vi "Live_ConvertSettings_Example_IMAQ.vi"() -> ()   [LabVIEW 2019]
doc: "This example demonstrates the image acquisition with one camera in ring buffer mode together with a live display of the latest images during record. After record is stopped, the images can be addressed by index.\nAdditionally the image convert settings can be adjusted at any time\nNote that this example will not be fail save, i.e. doesnt react on errors, just handles them forward to the end\n\nUsage:\nSelect your required image count and the camera setup before you start the program.\nOnce started, the camera class will be initialized and images will be recorded and displayed automatically\nYou can stop the images by pressing stop record.\nAfter stopped, the image at the selected index will be read out\nTo finish the program click on quit application, this will force an exit of the camera class\nYou can change your required ROI after and also during the record."
uses:
  camera/Camera.lvclass
  pco.sdk/TimingControl/TimingControl.lvlib
panel:
  in  "settingsChanged":bool
  in  "Trigger":bool
  in  "LUT File":path
  in  "data_format":T1(ring)=enum."RGBA8"
  out "Image":T2(plugin-control)
  in  "Auto Range":bool
  out "rawImage":u16[][](array[numeric])
  in  "iContrast [%]":i32 min=-100 max=99 step=1
  in  "Gamma":dbl=1.0 min=0.01 max=10.0 step=0.01 format="%.2f"
  in  "whiteBalance":bool
  in  "iScale_max":u16=60000 step=1
  in  "iScale_min":u16=200 step=1
  in  "Image Index":u32 max=9
  out "Recorded Images":u32
  in  "TriggerMode":T3(ring)
  in  "Quit":bool
  out "Error":errorcluster {"code" format="%x"}
  in  "Stop Record":bool
  out "Recording On":bool
  in  "cropY1":u64=2 min=1 max=2160 step=1
  in  "cropX1":u64=2 min=1 max=2560 step=1
  in  "cropY0":u64=1 min=1 max=2159 step=1
  in  "cropX0":u64=1 min=1 max=2559 step=1
  out "Image Height":u64
  out "Image Width":u64
  in  "dwImgCount":u32=10 caption="Required Number of Images" max=2397
  in  "Exposure Time [s]":dbl=0.010000000000000002 min=0.0005 max=2.0 step=0.001
  # "This example demonstrates the image acquisition with one camera in ring buffer mode together with a live display of the latest images during record. After record is stopped, the images can be addressed by index.\nAdditionally the image convert settings can be adjusted at any time\nNote that this example will not be fail save, i.e. doesnt react on errors, just handles them forward to the end\n\nUsage:\nSelect your required image count and the camera setup before you start the program.\nOnce started, the camera class will be initialized and images will be recorded and displayed automatically\nYou can stop the images by pressing stop record.\nAfter stopped, the image at the selected index will be read out\nTo finish the program click on quit application, this will force an exit of the camera class\nYou can change the cropped region after and also during the record."
  # "pco.labview"
  # "Camera Setup"
  # "Recording Control"
  # "Parameters for image readout"
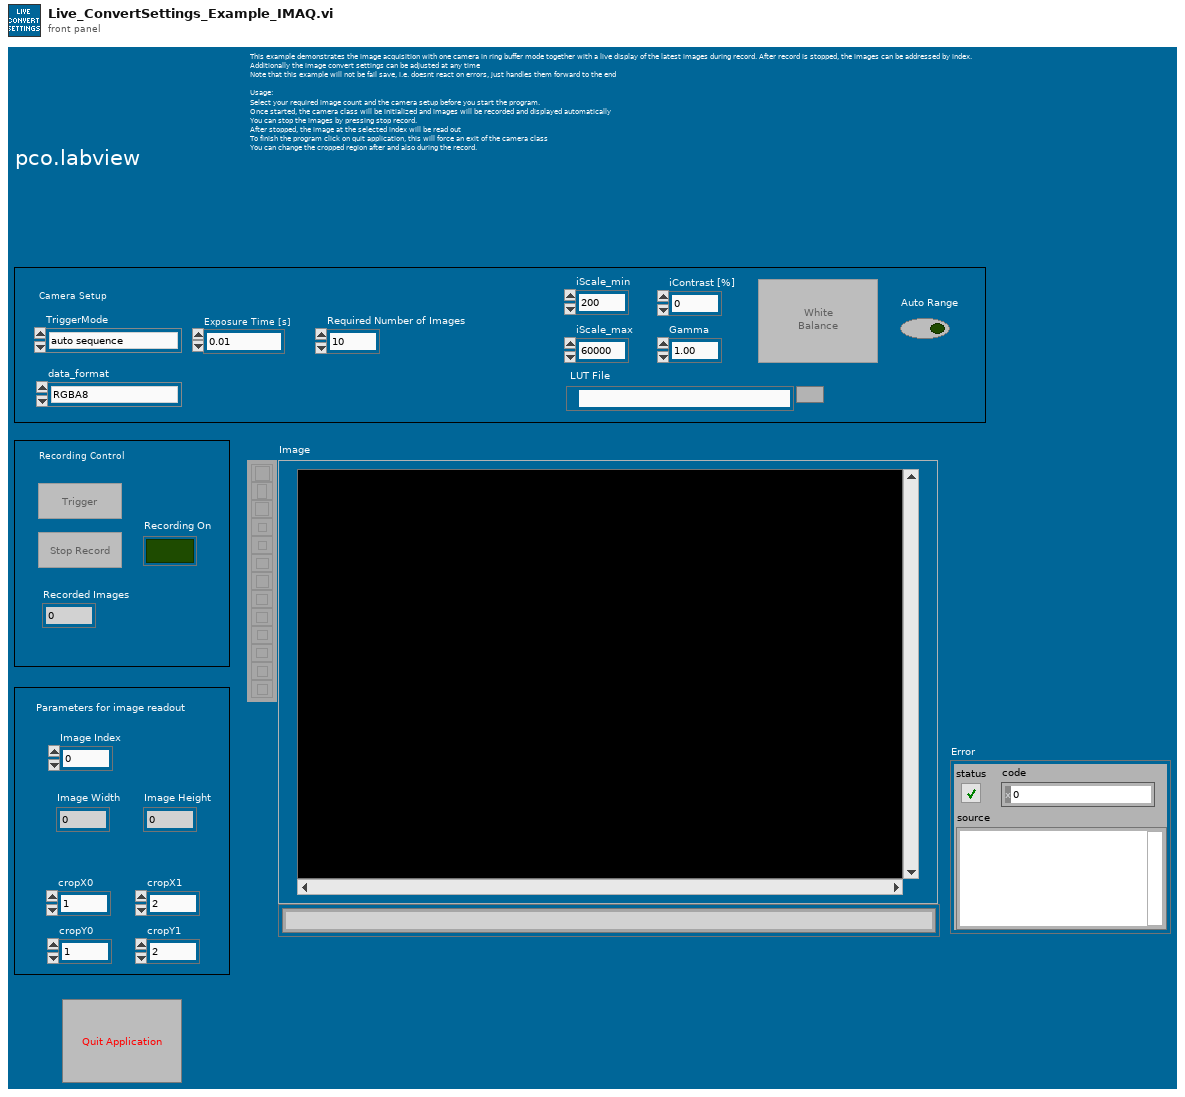
[diagram p1: front panel]
types:
  T1 = enum16{"Undefined", "Mono8", "Mono16", "BGRA8", "RGBA8", "BGRA16", "RGBA16", "CompressedMono8"}
  T2 = typedef "IMAQ Image.ctl" = refnum<image>
  T3 = enum16{"auto sequence", "software trigger", "external exposure start", "external exposure control"}
  T4 = enum16{"sequence", "sequence non blocking", "ring buffer", "fifo", "tif", "multitif", "pcoraw", "b16", "dicom", "multidicom", "camram_ring", "camram_segment"}
  T5 = enum8{"Enabled", "Disabled", "Disabled and Grayed Out"}
  T6 = cluster{"serial":u32, "type":u16, "sub_type":u16, "interface_type":u16, "bit_resolution":u16, "min_exposure_time_s":dbl, "max_exposure_time_s":dbl, "min_exposure_step_s":dbl, "min_delay_time_s":dbl, "max_delay_time_s":dbl, "min_delay_step_s":dbl, "min_width":u64, "min_height":u64, "max_width":u64, "max_height":u64, "roi_step_horz":u64, "roi_step_vert":u64, "roi_symmetric_horz":bool, "roi_symmetric_vert":bool, "has_timestamp_mode":bool, "has_timestamp_mode_ascii_only":bool, "pixelrate_vec":u32[], "conversion_factor_vec":sgl[], "has_trigger_mode_extexpctrl":bool, "has_acquire_mode":bool, "has_ext_acquire_mode":bool, "has_metadata_mode":bool, "has_ram":bool, "binning_horz_vec":u16[], "binning_vert_vec":u16[], "has_average_binning":bool, "pixel_format_vec":u32[]}
  T7 = typedef "Image Type" = u32
  T8 = cluster{"wSignalNum":u16, "wEnabled":u16, "wType":u16, "wPolarity":u16, "wFilterSetting":u16, "wSelected":u16, "dwParameter":u32[], "dwSignalFunctionality":u32[]}
  T9 = typedef "Camera.lvclass/binning.ctl" = cluster{"vert":u16, "horz":u16, "mode":u16}
  T10 = cluster{"exposure_time_s":dbl, "delay_time_s":dbl, "roi":cluster{"x0":u64, "y0":u64, "x1":u64, "y1":u64}, "timestamp_mode":u16, "pixelrate":u32, "conversion_factor":sgl, "trigger_mode":u16, "acquire_mode":u16, "acquire_sequence_number":u32, "metadata_mode":u16, "noisefilter_mode":u16, "pixel_format":u32, "binning":T9, "auto_exposure":cluster{"region":u16, "min_exposure_s":dbl, "max_exposure_s":dbl}}
  T11 = cluster{"sharpen":bool, "adaptive_sharpen":bool, "flip_vertical":bool, "auto_minmax":bool, "add_conv_flags":u32, "min_limit":u16, "max_limit":u16, "gamma":dbl, "contrast":i32, "pco_debayer_algorithm":bool, "color_temperature":i32, "color_saturation":i32, "color_vibrance":i32, "color_tint":i32, "lut_file":path}
  T12 = cluster{"Plane 4 (alpha)":u16, "Plane 1 (Red)":u16, "Plane 2 (Green)":u16, "Plane 3 (Blue)":u16}[][]
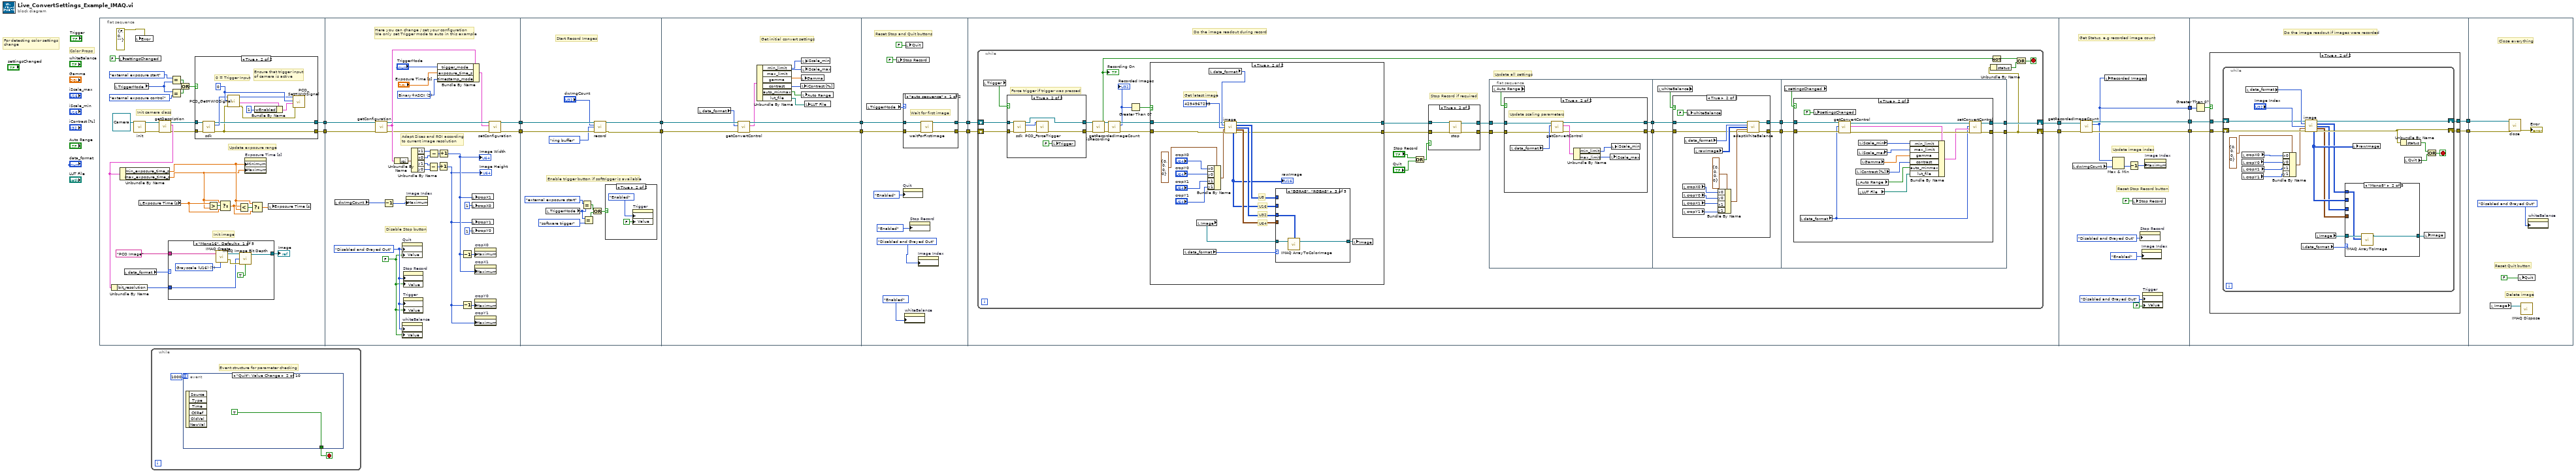
[diagram p0: block diagram]
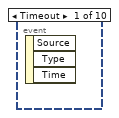
[diagram p2: hidden frame]
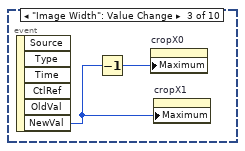
[diagram p3: hidden frame]
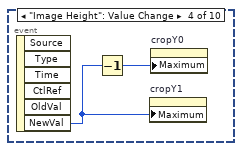
[diagram p4: hidden frame]
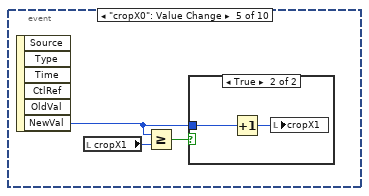
[diagram p5: hidden frame]
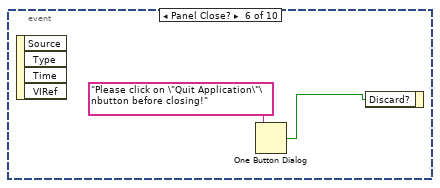
[diagram p7: hidden frame]
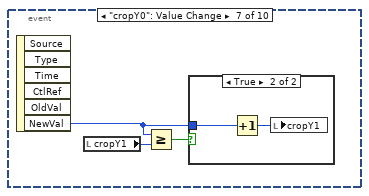
[diagram p8: hidden frame]
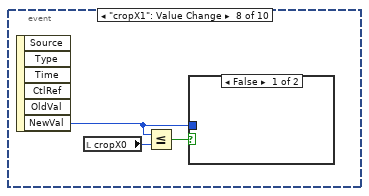
[diagram p10: hidden frame]
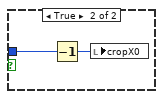
[diagram p11: hidden frame]
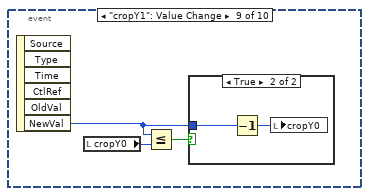
[diagram p12: hidden frame]
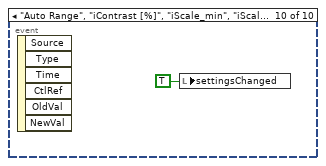
[diagram p14: hidden frame]
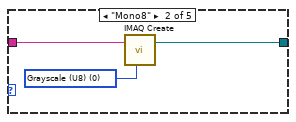
[diagram p16: hidden frame]
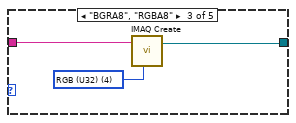
[diagram p17: hidden frame]
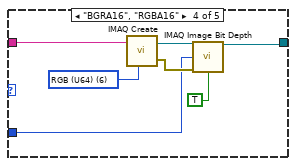
[diagram p18: hidden frame]
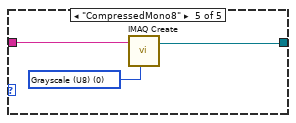
[diagram p19: hidden frame]
diagram:
  # "For detecting color settings\nchange"
  # "Color Props"
  n1 = flat-sequence {
    tunnel: [w24] -> w7
    tunnel: [w25] -> w1
    tunnel: [w85] -> w17
    tunnel: [w89] -> w16
    tunnel: w7 -> [w84]
    tunnel: w1 -> [w83]
    tunnel: w17 -> [w119]
    tunnel: w16 -> [w120]
    tunnel: [w116] -> w11
    tunnel: [w117] -> w8
    tunnel: w11 -> [w133]
    tunnel: [w128] -> w10
    tunnel: [w134] -> w9
    tunnel: w8 -> [w124]
    tunnel: w10 -> [w141]
    tunnel: w9 -> [w142]
    tunnel: [w140] -> w15
    tunnel: [w137] -> w3
    tunnel: w15 -> [w155]
    tunnel: [w154] -> w14
    tunnel: [w153] -> w6
    tunnel: w3 -> [w152]
    tunnel: w14 -> [w302]
    tunnel: [w300] -> w13
    tunnel: w6 -> [w295]
    tunnel: [w294] -> w5
    tunnel: [w293] -> w2
    tunnel: w13 -> [w311]
    tunnel: [w310] -> w12
    tunnel: w5 -> [w309]
    tunnel: [w308] -> w4
    tunnel: w2 -> [w306]
    tunnel: w12 -> [w359]
    tunnel: w4 -> [w356]
    frame #0 {
      # "Update exposure range"
      # "Init image"
      # "Init camera class"
      n2 = local read "TriggerMode"() -> (w18:T3)
      n3 = local write "settingsChanged"(FALSE ("settingsChanged")) -> ()
      n4 = local read "data_format"() -> (w31:T1)
      n5 = call-dynamic "init.vi"("Camera in"=refnum<class "Camera.lvclass"> refnum) -> ("Camera out"=w34:refnum<class "Camera.lvclass">, "error out"=w35:errorcluster)  [unwired: 8 in]
      n6 = local write "Error"(errorcluster {"status"=FALSE, "code"=0, "source"=""} ("error IO")) -> ()
      n7 = local read "Exposure Time [s]"() -> (w43:dbl)
      n8 = call-dynamic "getDescription.vi"("error in (no error)"=w35, "Camera in"=w34) -> ("error out"=w26:errorcluster, "description"=w29:T6, "Camera out"=w27:refnum<class "Camera.lvclass">)  [unwired: 7 in]
      n9 = Unbundle By Name(w29) -> ("bit_resolution"=w28:u16)
      n10 = Unbundle By Name(w29) -> ("min_exposure_time_s"=w33:dbl, "max_exposure_time_s"=w32:dbl)
      n11 = case shown="\"Mono16\", Default" w31 {
        tunnel: "PCO Image" ("Image Name") -> [w63 w67 w69 w76 w79]
        tunnel: [w59 w65 w68 w72 w78] -> w36
        tunnel: w28 -> [w58 _ _ w71 _]
        frame "Mono16", Default {
          w64 = T7 7 items=["Grayscale (U8)", "Grayscale (I16)", "Grayscale (SGL)", "Complex (CSG)", "RGB (U32)", "HSL (U32)", "RGB (U64)", "Grayscale (U16)"] ("Image Type")
          n12 = call "IMAQ Create"("Image Name"=w63, "Image Type"=w64) -> ("New Image"=w61:T2, "error out"=w60:errorcluster)  [unwired: 3 in]
          n13 = call "IMAQ Image Bit Depth"("Image"=w61, "Bit Depth (0)"=w58, "error in (no error)"=w60, "Get/Set Bit Depth? (Set)"=TRUE) -> ("Image Out"=w59:T2)  [unwired: 9 in, 2 out]
        }
        frame "Mono8" {
          w66 = T7 0 items=["Grayscale (U8)", "Grayscale (I16)", "Grayscale (SGL)", "Complex (CSG)", "RGB (U32)", "HSL (U32)", "RGB (U64)", "Grayscale (U16)"] ("Image Type")
          n14 = call "IMAQ Create"("Image Name"=w67, "Image Type"=w66) -> ("New Image"=w65:T2)  [unwired: 3 in, 1 out]
        }
        frame "BGRA8", "RGBA8" {
          w70 = T7 4 items=["Grayscale (U8)", "Grayscale (I16)", "Grayscale (SGL)", "Complex (CSG)", "RGB (U32)", "HSL (U32)", "RGB (U64)", "Grayscale (U16)"] ("Image Type")
          n15 = call "IMAQ Create"("Image Name"=w69, "Image Type"=w70) -> ("New Image"=w68:T2)  [unwired: 3 in, 1 out]
        }
        frame "BGRA16", "RGBA16" {
          w77 = T7 6 items=["Grayscale (U8)", "Grayscale (I16)", "Grayscale (SGL)", "Complex (CSG)", "RGB (U32)", "HSL (U32)", "RGB (U64)", "Grayscale (U16)"] ("Image Type")
          n16 = call "IMAQ Create"("Image Name"=w76, "Image Type"=w77) -> ("New Image"=w74:T2, "error out"=w73:errorcluster)  [unwired: 3 in]
          n17 = call "IMAQ Image Bit Depth"("Image"=w74, "Bit Depth (0)"=w71, "error in (no error)"=w73, "Get/Set Bit Depth? (Set)"=TRUE) -> ("Image Out"=w72:T2)  [unwired: 9 in, 2 out]
        }
        frame "CompressedMono8" {
          w80 = T7 0 items=["Grayscale (U8)", "Grayscale (I16)", "Grayscale (SGL)", "Complex (CSG)", "RGB (U32)", "HSL (U32)", "RGB (U64)", "Grayscale (U16)"] ("Image Type")
          n18 = call "IMAQ Create"("Image Name"=w79, "Image Type"=w80) -> ("New Image"=w78:T2)  [unwired: 3 in, 1 out]
        }
      }
      "Image" <- w36
      n19 = Equal?(x=T3."external exposure start" ("TriggerMode"), y=w18) -> (x = y?=w22:bool)
      n20 = Equal?(x=w18, y=T3."external exposure control" ("TriggerMode")) -> (x = y?=w21:bool)
      n21 = Or(x=w22, y=w21) -> (x .or. y?=w20:bool)
      n22 = case shown="True" w20 {
        tunnel: w27 -> [w46 w50]
        tunnel: w26 -> [w45 w49]
        tunnel: [w45 w47] -> w25
        tunnel: [w46 w48] -> w24
        frame False {
        }
        frame True {
          w55 = u16 0 ("wSignalNum")
          # "0 = Trigger Input"
          # "Ensure that trigger input\nof camera is active"
          n23 = call-dynamic "sdk.vi"("Camera in"=w50, "error in (no error)"=w49) -> ("Camera out"=w48:refnum<class "Camera.lvclass">, "sdk"=w51:u64, "error out"=w47:errorcluster)  [unwired: 11 in]
          n24 = call "PCO_GetHWIOSignal.vi"("error in (no error)"=w47, "wSignalNum"=w55, "ph"=w51) -> ("error out"=w53:errorcluster, "strSignal"=w57:T8, "ph out"=w52:u64)  [unwired: 5 in, 1 out]
          n25 = Bundle By Name(cluster=w57, "wEnabled"=u16 1) -> (w54:T8)
          n26 = call "PCO_SetHWIOSignal.vi"("error in (no error)"=w53, "strSignal"=w54, "wSignalNum"=w55, "ph"=w52) -> ()  [unwired: 5 in, 3 out]
        }
      }
      n27 = Greater?(x=w43, y=w32) -> (0:w44:bool)
      n28 = Select(t=w32, s=w44, f=w43) -> (s? t:f=w41:dbl)
      n29 = Less?(x=w41, y=w33) -> (x < y?=w42:bool)
      n30 = property on="Exposure Time [s]" class="DigNum (strict)"("Minimum"=w33, "Maximum"=w32) -> ()  [unwired: 2 in, 2 out]
      n31 = Select(t=w33, s=w42, f=w41) -> (s? t:f=w40:dbl)
      n32 = local write "Exposure Time [s]"(w40) -> ()
    }
    frame #1 {
      w95 = u16 2 items=["OFF", "Binary", "Binary+ASCII", "ASCII"] ("wTimeStampMode")
      w81 = FALSE ("Stop")
      w82 = T5."Disabled and Grayed Out" ("Disabled")
      # "Disable Stop button"
      # "Adapt Sizes and ROI according\nto current image resolution"
      # "Here you can change / set your configuration\nWe only set Trigger mode to auto in this example"
      n33 = local read "dwImgCount"() -> (w96:u32)
      n34 = call-dynamic "getConfiguration.vi"("error in (no error)"=w83, "Camera in"=w84) -> ("error out"=w90:errorcluster, "configuration"=w101:T10, "Camera out"=w92:refnum<class "Camera.lvclass">)  [unwired: 7 in]
      n35 = Decrement(x=w96) -> (x-1=w86:u32)
      n36 = Unbundle By Name(w101) -> ("roi"=w102:cluster{"x0":u64, "y0":u64, "x1":u64, "y1":u64})
      n37 = property on="Quit" class="Bool (strict)"("DisabledEnum"=w82, "Value"=w81) -> ()  [unwired: 2 in, 2 out]
      n38 = property on="whiteBalance" class="Bool (strict)"("DisabledEnum"=w82, "Value"=w81) -> ()  [unwired: 2 in, 2 out]
      n39 = property on="Stop Record" class="Bool (strict)"("DisabledEnum"=w82, "Value"=w81) -> ()  [unwired: 2 in, 2 out]
      n40 = property on="Trigger" class="Bool (strict)"("DisabledEnum"=w82, "Value"=w81) -> ()  [unwired: 2 in, 2 out]
      n41 = property on="Image Index" class="DigNum (strict)"("Maximum"=w86) -> ()  [unwired: 2 in, 2 out]
      n42 = Unbundle By Name(w102) -> ("x1"=w104:u64, "x0"=w103:u64, "y1"=w106:u64, "y0"=w105:u64)
      n43 = Subtract(x=w106, y=w105) -> (x-y=w108:u64)
      n44 = Subtract(x=w104, y=w103) -> (x-y=w107:u64)
      n45 = Bundle By Name(cluster=w101, "trigger_mode"="TriggerMode", "exposure_time_s"="Exposure Time [s]", "timestamp_mode"=w95) -> (w91:T10)
      n46 = Increment(x=w108) -> (x+1=w87:u64)
      "Image Height" <- w87
      n47 = Increment(x=w107) -> (x+1=w88:u64)
      "Image Width" <- w88
      n48 = Decrement(x=w88) -> (x-1=w99:u64)
      n49 = Decrement(x=w87) -> (x-1=w100:u64)
      n50 = local write "cropX1"(w88) -> ()
      n51 = local write "cropX0"(u64 1 ("roiY0")) -> ()
      n52 = local write "cropY1"(w87) -> ()
      n53 = local write "cropY0"(u64 1 ("roiY0")) -> ()
      n54 = property on="cropX0" class="DigNum (strict)"("Maximum"=w99) -> ()  [unwired: 2 in, 2 out]
      n55 = property on="cropX1" class="DigNum (strict)"("Maximum"=w88) -> ()  [unwired: 2 in, 2 out]
      n56 = property on="cropY0" class="DigNum (strict)"("Maximum"=w100) -> ()  [unwired: 2 in, 2 out]
      n57 = property on="cropY1" class="DigNum (strict)"("Maximum"=w87) -> ()  [unwired: 2 in, 2 out]
      n58 = call-dynamic "setConfiguration.vi"("error in (no error)"=w90, "configuration"=w91, "Camera in"=w92) -> ("error out"=w89:errorcluster, "Camera out"=w85:refnum<class "Camera.lvclass">)  [unwired: 7 in]
    }
    frame #2 {
      # "Enable trigger button if softtrigger is available"
      # "Start Record Images"
      n59 = local read "TriggerMode"() -> (w114:T3)
      n60 = Equal?(x=T3."external exposure start" ("TriggerMode"), y=w114) -> (x = y?=w111:bool)
      n61 = Equal?(x=w114, y=T3."software trigger" ("TriggerMode")) -> (x = y?=w110:bool)
      n62 = Or(x=w111, y=w110) -> (x .or. y?=w112:bool)
      n63 = call-dynamic "record.vi"("Camera in"=w119, "num_images"="dwImgCount", "record_mode"=T4."ring buffer", "error in (no error)"=w120) -> ("Camera out"=w117:refnum<class "Camera.lvclass">, "error out"=w116:errorcluster)  [unwired: 10 in]
      n64 = case shown="True" w112 {
        frame False {
        }
        frame True {
          n65 = property on="Trigger" class="Bool (strict)"("DisabledEnum"=T5."Enabled" ("Disabled"), "Value"=FALSE ("Trigger")) -> ()  [unwired: 2 in, 2 out]
        }
      }
    }
    frame #3 {
      # "Get initial convert settings"
      n66 = local read "data_format"() -> (w123:T1)
      n67 = call-dynamic "getConvertControl.vi"("error in (no error)"=w133, "data_format"=w123, "Camera in"=w124) -> ("error out"=w128:errorcluster, "convert_control"=w132:T11, "Camera out"=w134:refnum<class "Camera.lvclass">)  [unwired: 6 in]
      n68 = Unbundle By Name(w132) -> ("min_limit"=w130:u16, "max_limit"=w129:u16, "gamma"=w131:dbl, "contrast"=w127:i32, "auto_minmax"=w126:bool, "lut_file"=w125:path)
      n69 = local write "iContrast [%]"(w127) -> ()
      n70 = local write "Gamma"(w131) -> ()
      n71 = local write "iScale_min"(w130) -> ()
      n72 = local write "iScale_max"(w129) -> ()
      n73 = local write "Auto Range"(w126) -> ()
      n74 = local write "LUT File"(w125) -> ()
    }
    frame #4 {
      # "Reset Stop and Quit buttons"
      n75 = local read "TriggerMode"() -> (w135:T3)
      n76 = local write "Stop Record"(FALSE ("Stop Record")) -> ()
      n77 = case shown="\"auto sequence\"" w135 {
        tunnel: w142 -> [w149 w151]
        tunnel: w141 -> [w148 w150]
        tunnel: [w147 w150] -> w140
        tunnel: [w146 w151] -> w137
        frame "auto sequence" {
          # "Wait for first image"
          n78 = call-dynamic "waitForFirstImage.vi"("error in (no error)"=w148, "Camera in"=w149) -> ("error out"=w147:errorcluster, "Camera out"=w146:refnum<class "Camera.lvclass">)  [unwired: 8 in]
        }
        frame Default {
          # "Don't wait \nif we trigger"
        }
      }
      n79 = property on="Quit" class="Bool (strict)"("DisabledEnum"=T5."Enabled" ("Disabled")) -> ()  [unwired: 2 in, 2 out]
      n80 = property on="whiteBalance" class="Bool (strict)"("DisabledEnum"=T5."Enabled" ("Disabled")) -> ()  [unwired: 2 in, 2 out]
      n81 = local write "Quit"(FALSE ("Stop")) -> ()
      n82 = property on="Stop Record" class="Bool (strict)"("DisabledEnum"=T5."Enabled" ("Disabled")) -> ()  [unwired: 2 in, 2 out]
      n83 = property on="Image Index" class="DigNum (strict)"("DisabledEnum"=T5."Disabled and Grayed Out" ("Disabled")) -> ()  [unwired: 2 in, 2 out]
    }
    frame #5 {
      # "Do the image readout during record"
      n84 = while {
        shift-right: [w165] -> w154
        shift-left: w155 -> [w168]
        shift-right: [w171] -> w153
        shift-left: w152 -> [w169]
        stop <- w183 stop-if-true
        # "Stop Record if required"
        # "Force trigger if trigger was pressed"
        # "Update all settings"
        n85 = local read "Trigger"() -> (w170:bool)
        n86 = case shown="True" w170 {
          tunnel: w169 -> [w227 w232]
          tunnel: w168 -> [w226 w231]
          tunnel: [w227 w230] -> w167
          tunnel: [w226 w229] -> w166
          frame False {
          }
          frame True {
            n87 = call-dynamic "sdk.vi"("Camera in"=w232, "error in (no error)"=w231) -> ("Camera out"=w230:refnum<class "Camera.lvclass">, "sdk"=w233:u64, "error out"=w234:errorcluster)  [unwired: 11 in]
            n88 = call "PCO_ForceTrigger.vi"("error in (no error)"=w234, "ph"=w233) -> ("error out"=w229:errorcluster)  [unwired: 6 in, 3 out]
            n89 = local write "Trigger"(FALSE ("Trigger")) -> ()
          }
        }
        n90 = call-dynamic "isRecording.vi"("Camera in"=w167, "error in (no error)"=w166) -> ("Camera out"=w179:refnum<class "Camera.lvclass">, "recording"=w181:bool, "error out"=w178:errorcluster)  [unwired: 11 in]
        "Recording On" <- w181
        n91 = call-dynamic "getRecordedImageCount.vi"("Camera in"=w179, "error in (no error)"=w178) -> ("Camera out"=w176:refnum<class "Camera.lvclass">, "recorded_image_count"=w164:u32, "error out"=w177:errorcluster)  [unwired: 11 in]
        "Recorded Images" <- w164
        n92 = Greater Than 0?(x=w164) -> (x > 0?=w163:bool)
        n93 = case shown="True" w163 {
          tunnel: w177 -> [w190 w203]
          tunnel: w176 -> [w191 w194]
          tunnel: [w190 w192] -> w159
          tunnel: [w191 w193] -> w158
          frame False {
          }
          frame True {
            # "U64"
            # "U32"
            # "U8"
            # "U16"
            # "Get latest image"
            n94 = local read "data_format"() -> (w195:T1)
            n95 = local read "Image"() -> (w200:T2)
            n96 = Bundle By Name(cluster=cluster{"x0":u64, "y0":u64, "x1":u64, "y1":u64} {"x0"=0, "y0"=0, "x1"=0, "y1"=0} ("roi"), "x0"="cropX0", "y0"="cropY0", "x1"="cropX1", "y1"="cropY1") -> (w206:cluster{"x0":u64, "y0":u64, "x1":u64, "y1":u64})
            n97 = local read "data_format"() -> (w202:T1)
            n98 = call-dynamic "image.vi"("Camera in"=w194, "data_format"=w202, "image_index"=u32 4294967295 ("dwImgIdx"), "crop"=w206, "error in (no error)"=w203) -> ("Camera out"=w193:refnum<class "Camera.lvclass">, "image (U8)"=w197:u8[][], "image (U32)"=w198:u32[][], "image (U64)"=w199:T12, "raw_image (U16)"=w196:u16[][], "error out"=w192:errorcluster)  [unwired: 2 in, 3 out]
            "rawImage" <- w196
            n99 = case shown="\"BGRA8\", \"RGBA8\"" w195 {
              tunnel: w200 -> [w213 w216 w219 w222 w225]
              tunnel: [w211 w214 w218 w220 w224] -> w201
              tunnel: w199 -> [_ _ _ w221 _]
              tunnel: w198 -> [_ _ w217 _ _]
              tunnel: w197 -> [_ w215 _ _ w223]
              tunnel: w196 -> [w212 _ _ _ _]
              frame "Mono16", Default {
                n100 = call "IMAQ ArrayToImage"("Image Pixels (U16)"=w212, "Image"=w213) -> ("Image Out"=w211:T2)  [unwired: 8 in, 1 out]
              }
              frame "Mono8" {
                n101 = call "IMAQ ArrayToImage"("Image Pixels (U8)"=w215, "Image"=w216) -> ("Image Out"=w214:T2)  [unwired: 8 in, 1 out]
              }
              frame "BGRA8", "RGBA8" {
                n102 = call "IMAQ ArrayToColorImage"("Image Pixels (U32)"=w217, "Image"=w219) -> ("Image Out"=w218:T2)  [unwired: 3 in, 1 out]
              }
              frame "BGRA16", "RGBA16" {
                n103 = call "IMAQ ArrayToColorImage"("Image"=w222, "Image Pixels (U64)"=w221) -> ("Image Out"=w220:T2)  [unwired: 3 in, 1 out]
              }
              frame "CompressedMono8" {
                n104 = call "IMAQ ArrayToImage"("Image Pixels (U8)"=w223, "Image"=w225) -> ("Image Out"=w224:T2)  [unwired: 8 in, 1 out]
              }
            }
            n105 = local write "Image"(w201) -> ()
          }
        }
        n106 = Or(x="Stop Record", y="Quit") -> (x .or. y?=w162:bool)
        n107 = case shown="True" w162 {
          tunnel: w159 -> [w185 w186]
          tunnel: [w184 w188] -> w157
          tunnel: [w185 w189] -> w156
          tunnel: w158 -> [w184 w187]
          frame False {
          }
          frame True {
            n108 = call-dynamic "stop.vi"("error in (no error)"=w186, "Camera in"=w187) -> ("error out"=w189:errorcluster, "Camera out"=w188:refnum<class "Camera.lvclass">)  [unwired: 8 in]
          }
        }
        n109 = flat-sequence {
          tunnel: w156 -> [w237]
          tunnel: w157 -> [w238]
          tunnel: [w236] -> w175
          tunnel: [w235] -> w174
          tunnel: w175 -> [w253]
          tunnel: w174 -> [w252]
          tunnel: [w251] -> w173
          tunnel: [w250] -> w172
          tunnel: w173 -> [w272]
          tunnel: w172 -> [w273]
          tunnel: [w271] -> w165
          tunnel: [w270] -> w171
          frame #0 {
            n110 = local read "Auto Range"() -> (w239:bool)
            n111 = case shown="True" w239 {
              tunnel: w238 -> [w241 w245]
              tunnel: w237 -> [w240 w244]
              tunnel: [w240 w243] -> w236
              tunnel: [w241 w242] -> w235
              frame False {
              }
              frame True {
                # "Update scaling parameters"
                n112 = local read "data_format"() -> (w249:T1)
                n113 = call-dynamic "getConvertControl.vi"("error in (no error)"=w244, "data_format"=w249, "Camera in"=w245) -> ("error out"=w243:errorcluster, "convert_control"=w246:T11, "Camera out"=w242:refnum<class "Camera.lvclass">)  [unwired: 6 in]
                n114 = Unbundle By Name(w246) -> ("min_limit"=w247:u16, "max_limit"=w248:u16)
                n115 = local write "iScale_max"(w248) -> ()
                n116 = local write "iScale_min"(w247) -> ()
              }
            }
          }
          frame #1 {
            n117 = local read "whiteBalance"() -> (w254:bool)
            n118 = case shown="True" w254 {
              tunnel: w253 -> [w255 w261]
              tunnel: w252 -> [w256 w260]
              tunnel: [w255 w259] -> w251
              tunnel: [w256 w258] -> w250
              frame False {
              }
              frame True {
                n119 = local read "cropX0"() -> (w266:u64)
                n120 = local read "cropY0"() -> (w265:u64)
                n121 = local read "cropX1"() -> (w264:u64)
                n122 = local read "cropY1"() -> (w257:u64)
                n123 = local read "data_format"() -> (w268:T1)
                n124 = local write "whiteBalance"(FALSE ("whiteBalance")) -> ()
                n125 = local read "rawImage"() -> (w267:u16[][])
                n126 = Bundle By Name(cluster=cluster{"x0":u64, "y0":u64, "x1":u64, "y1":u64} {"x0"=0, "y0"=0, "x1"=0, "y1"=0} ("roi"), "x0"=w266, "y0"=w265, "x1"=w264, "y1"=w257) -> (w263:cluster{"x0":u64, "y0":u64, "x1":u64, "y1":u64})
                n127 = call-dynamic "adaptWhiteBalance.vi"("Camera in"=w260, "data_format"=w268, "raw_image (U16)"=w267, "roi"=w263, "error in (no error)"=w261) -> ("Camera out"=w258:refnum<class "Camera.lvclass">, "error out"=w259:errorcluster)  [unwired: 9 in]
              }
            }
          }
          frame #2 {
            n128 = local read "settingsChanged"() -> (w274:bool)
            n129 = case shown="True" w274 {
              tunnel: w273 -> [w276 w282]
              tunnel: w272 -> [w275 w281]
              tunnel: [w275 w278] -> w271
              tunnel: [w276 w277] -> w270
              frame False {
              }
              frame True {
                n130 = local read "data_format"() -> (w280:T1)
                n131 = local write "settingsChanged"(FALSE ("whiteBalance")) -> ()
                n132 = call-dynamic "getConvertControl.vi"("error in (no error)"=w281, "data_format"=w280, "Camera in"=w282) -> ("error out"=w284:errorcluster, "convert_control"=w291:T11, "Camera out"=w285:refnum<class "Camera.lvclass">)  [unwired: 6 in]
                n133 = local read "iContrast [%]"() -> (w287:i32)
                n134 = local read "Auto Range"() -> (w286:bool)
                n135 = local read "iScale_max"() -> (w289:u16)
                n136 = local read "iScale_min"() -> (w290:u16)
                n137 = local read "LUT File"() -> (w279:path)
                n138 = local read "Gamma"() -> (w288:dbl)
                n139 = Bundle By Name(cluster=w291, "min_limit"=w290, "max_limit"=w289, "gamma"=w288, "contrast"=w287, "auto_minmax"=w286, "lut_file"=w279) -> (w283:T11)
                n140 = call-dynamic "setConvertControl.vi"("error in (no error)"=w284, "convert_control"=w283, "data_format"=w280, "Camera in"=w285) -> ("error out"=w278:errorcluster, "Camera out"=w277:refnum<class "Camera.lvclass">)  [unwired: 6 in]
              }
            }
          }
        }
        n141 = Unbundle By Name(w165) -> ("status"=w182:bool)
        n142 = Not(x=w181) -> (.not. x?=w180:bool)
        n143 = Or(x=w180, y=w182) -> (x .or. y?=w183:bool)
      }
    }
    frame #6 {
      # "Update image index"
      # "Reset Stop Record button"
      # "Get Status, e.g recorded image count"
      n144 = local read "dwImgCount"() -> (w301:u32)
      n145 = call-dynamic "getRecordedImageCount.vi"("Camera in"=w295, "error in (no error)"=w302) -> ("Camera out"=w294:refnum<class "Camera.lvclass">, "recorded_image_count"=w293:u32, "error out"=w300:errorcluster)  [unwired: 11 in]
      n146 = local write "Recorded Images"(w293) -> ()
      n147 = Max & Min(x=w293, y=w301) -> (min(x,y)=w303:u32)  [unwired: 1 out]
      n148 = Decrement(x=w303) -> (x-1=w298:u32)
      n149 = local write "Stop Record"(FALSE ("Stop Record")) -> ()
      n150 = property on="Stop Record" class="Bool (strict)"("DisabledEnum"=T5."Disabled and Grayed Out" ("Disabled")) -> ()  [unwired: 2 in, 2 out]
      n151 = property on="Image Index" class="DigNum (strict)"("DisabledEnum"=T5."Enabled" ("Disabled")) -> ()  [unwired: 2 in, 2 out]
      n152 = property on="Trigger" class="Bool (strict)"("DisabledEnum"=T5."Disabled and Grayed Out" ("Disabled"), "Value"=FALSE ("Trigger")) -> ()  [unwired: 2 in, 2 out]
      n153 = property on="Image Index" class="DigNum (strict)"("Maximum"=w298) -> ()  [unwired: 2 in, 2 out]
    }
    frame #7 {
      # "Do the image readout if images were recorded"
      n154 = Greater Than 0?(x=w306) -> (x > 0?=w307:bool)
      n155 = case shown="True" w307 {
        tunnel: w311 -> [w312 w317]
        tunnel: [w312 w316] -> w310
        tunnel: w309 -> [w313 w315]
        tunnel: [w313 w314] -> w308
        frame False {
        }
        frame True {
          n156 = while {
            shift-right: [w331] -> w316
            shift-left: w317 -> [w339]
            shift-right: [w318] -> w314
            shift-left: w315 -> [w319]
            stop <- w333 stop-if-true
            n157 = local read "cropX0"() -> (w329:u64)
            n158 = local read "cropY0"() -> (w330:u64)
            n159 = local read "cropX1"() -> (w337:u64)
            n160 = local read "cropY1"() -> (w336:u64)
            n161 = local read "data_format"() -> (w327:T1)
            n162 = Bundle By Name(cluster=cluster{"x0":u64, "y0":u64, "x1":u64, "y1":u64} {"x0"=0, "y0"=0, "x1"=0, "y1"=0} ("roi"), "x0"=w329, "y0"=w330, "x1"=w337, "y1"=w336) -> (w338:cluster{"x0":u64, "y0":u64, "x1":u64, "y1":u64})
            n163 = local read "data_format"() -> (w320:T1)
            n164 = call-dynamic "image.vi"("Camera in"=w319, "data_format"=w327, "image_index"="Image Index", "crop"=w338, "error in (no error)"=w339) -> ("Camera out"=w318:refnum<class "Camera.lvclass">, "image (U8)"=w323:u8[][], "image (U32)"=w322:u32[][], "image (U64)"=w321:T12, "raw_image (U16)"=w324:u16[][], "error out"=w331:errorcluster)  [unwired: 2 in, 3 out]
            n165 = local read "Image"() -> (w325:T2)
            n166 = case shown="\"Mono8\"" w320 {
              tunnel: w325 -> [w342 w345 w348 w351 w354]
              tunnel: [w340 w343 w347 w349 w353] -> w326
              tunnel: w321 -> [_ _ _ w350 _]
              tunnel: w322 -> [_ _ w346 _ _]
              tunnel: w323 -> [_ w344 _ _ w352]
              tunnel: w324 -> [w341 _ _ _ _]
              frame "Mono16", Default {
                n167 = call "IMAQ ArrayToImage"("Image Pixels (U16)"=w341, "Image"=w342) -> ("Image Out"=w340:T2)  [unwired: 8 in, 1 out]
              }
              frame "Mono8" {
                n168 = call "IMAQ ArrayToImage"("Image Pixels (U8)"=w344, "Image"=w345) -> ("Image Out"=w343:T2)  [unwired: 8 in, 1 out]
              }
              frame "BGRA8", "RGBA8" {
                n169 = call "IMAQ ArrayToColorImage"("Image Pixels (U32)"=w346, "Image"=w348) -> ("Image Out"=w347:T2)  [unwired: 3 in, 1 out]
              }
              frame "BGRA16", "RGBA16" {
                n170 = call "IMAQ ArrayToColorImage"("Image"=w351, "Image Pixels (U64)"=w350) -> ("Image Out"=w349:T2)  [unwired: 3 in, 1 out]
              }
              frame "CompressedMono8" {
                n171 = call "IMAQ ArrayToImage"("Image Pixels (U8)"=w352, "Image"=w354) -> ("Image Out"=w353:T2)  [unwired: 8 in, 1 out]
              }
            }
            n172 = local write "rawImage"(w324) -> ()
            n173 = Unbundle By Name(w331) -> ("status"=w334:bool)
            n174 = local read "Quit"() -> (w335:bool)
            n175 = local write "Image"(w326) -> ()
            n176 = Or(x=w334, y=w335) -> (x .or. y?=w333:bool)
          }
        }
      }
    }
    frame #8 {
      # "Delete image"
      # "Close everything"
      # "Reset Quit button"
      n177 = local read "Image"() -> (w355:T2)
      n178 = call-dynamic "close.vi"("error in (no error)"=w359, "Camera in"=w356) -> ("error out"=→"Error":errorcluster)  [unwired: 9 in]
      n179 = local write "Quit"(FALSE ("Stop Record")) -> ()
      n180 = call "IMAQ Dispose"("Image"=w355) -> ()  [unwired: 5 in, 1 out]
      n181 = property on="whiteBalance" class="Bool (strict)"("DisabledEnum"=T5."Disabled and Grayed Out" ("Disabled")) -> ()  [unwired: 2 in, 2 out]
    }
  }
  n182 = while {
    stop <- w361 stop-if-true
    # "Event structure for parameter checking"
    n183 = event shown="[1] \"Quit\": Value Change" {
      selector: _ -> [_ _ _ _ _ _ _ _ _ _]
      dyn-events: _ -> [_ _ _ _ _ _ _ _ _ _]
      timeout: 1000 -> [_ _ _ _ _ _ _ _ _ _]
      tunnel: [_ TRUE _ _ _ _ _ _ _ _] -> w361
      event Timeout {
        n184 = event-data() -> ()  [unwired: 1 in, 3 out]
      }
      event "Quit": Value Change {
        n185 = event-data() -> ()  [unwired: 1 in, 6 out]
      }
      event "Image Width": Value Change {
        n186 = event-data() -> ("NewVal"=w364:u64)  [unwired: 1 in, 5 out]
        n187 = Decrement(x=w364) -> (x-1=w365:u64)
        n188 = property on="cropX0" class="DigNum (strict)"("Maximum"=w365) -> ()  [unwired: 2 in, 2 out]
        n189 = property on="cropX1" class="DigNum (strict)"("Maximum"=w364) -> ()  [unwired: 2 in, 2 out]
      }
      event "Image Height": Value Change {
        n190 = event-data() -> ("NewVal"=w366:u64)  [unwired: 1 in, 5 out]
        n191 = Decrement(x=w366) -> (x-1=w367:u64)
        n192 = property on="cropY1" class="DigNum (strict)"("Maximum"=w366) -> ()  [unwired: 2 in, 2 out]
        n193 = property on="cropY0" class="DigNum (strict)"("Maximum"=w367) -> ()  [unwired: 2 in, 2 out]
      }
      event "cropX0": Value Change {
        n194 = event-data() -> ("NewVal"=w368:u64)  [unwired: 1 in, 5 out]
        n195 = local read "cropX1"() -> (w370:u64)
        n196 = Greater Or Equal?(x=w368, y=w370) -> (x >= y?=w369:bool)
        n197 = case shown="True" w369 {
          tunnel: w368 -> [_ w372]
          frame False {
          }
          frame True {
            n198 = Increment(x=w372) -> (x+1=w371:u64)
            n199 = local write "cropX1"(w371) -> ()
          }
        }
      }
      event Panel Close? {
        n200 = event-data() -> ()  [unwired: 1 in, 4 out]
        n201 = One Button Dialog(message="Please click on \"Quit Application\"\nbutton before closing!") -> (true=w373:bool)  [unwired: 1 in]
        n202 = event-data("Discard?"=w373) -> ()  [unwired: 1 in, 1 out]
      }
      event "cropY0": Value Change {
        n203 = event-data() -> ("NewVal"=w375:u64)  [unwired: 1 in, 5 out]
        n204 = local read "cropY1"() -> (w377:u64)
        n205 = Greater Or Equal?(x=w375, y=w377) -> (x >= y?=w376:bool)
        n206 = case shown="True" w376 {
          tunnel: w375 -> [_ w379]
          frame False {
          }
          frame True {
            n207 = Increment(x=w379) -> (x+1=w378:u64)
            n208 = local write "cropY1"(w378) -> ()
          }
        }
      }
      event "cropX1": Value Change {
        n209 = event-data() -> ("NewVal"=w380:u64)  [unwired: 1 in, 5 out]
        n210 = local read "cropX0"() -> (w382:u64)
        n211 = Less Or Equal?(x=w380, y=w382) -> (x <= y?=w381:bool)
        n212 = case shown="False" w381 {
          tunnel: w380 -> [_ w384]
          frame False {
          }
          frame True {
            n213 = Decrement(x=w384) -> (x-1=w383:u64)
            n214 = local write "cropX0"(w383) -> ()
          }
        }
      }
      event "cropY1": Value Change {
        n215 = event-data() -> ("NewVal"=w385:u64)  [unwired: 1 in, 5 out]
        n216 = local read "cropY0"() -> (w387:u64)
        n217 = Less Or Equal?(x=w385, y=w387) -> (x <= y?=w386:bool)
        n218 = case shown="True" w386 {
          tunnel: w385 -> [_ w389]
          frame False {
          }
          frame True {
            n219 = Decrement(x=w389) -> (x-1=w388:u64)
            n220 = local write "cropY0"(w388) -> ()
          }
        }
      }
      event "Auto Range", "iContrast [%]", "iScale_min", "iScale_max", "Gamma", "LUT File": Value Change {
        n221 = event-data() -> ()  [unwired: 1 in, 6 out]
        n222 = local write "settingsChanged"(TRUE ("settingsChanged")) -> ()
      }
    }
  }
